vi "Unidirectional Quadrature Decoder.vi"(10 "B":bool, 11 "A":bool) -> (3 "Counter":i32)   [LabVIEW 2018]
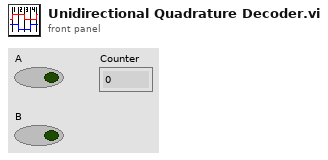
[diagram p1: front panel]
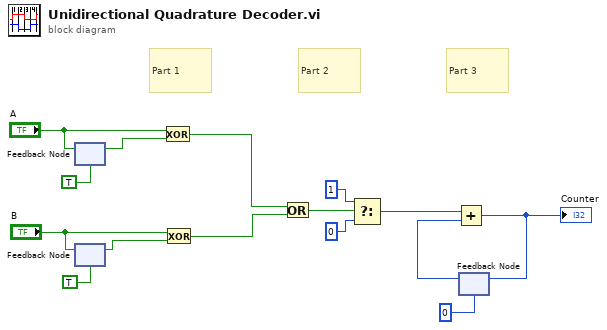
[diagram p0: block diagram]
diagram:
  # "Part 3"
  # "Part 2"
  # "Part 1"
  n1 = feedback-in #1("A") -> ()
  n2 = feedback #1(TRUE ("A")) -> (w7:bool)
  n3 = feedback #2(TRUE ("A")) -> (w5:bool)
  n4 = feedback-in #2("B") -> ()
  n5 = Exclusive Or(1:w7, 2:"A") -> (0:w15:bool)
  n6 = Exclusive Or(1:w5, 2:"B") -> (0:w14:bool)
  n7 = Or(x=w15, y=w14) -> (x .or. y?=w13:bool)
  n8 = Select(t=1, s=w13, f=0) -> (s? t:f=w9:i32)
  n9 = feedback #3(0) -> (w10:i32)
  n10 = Add(x=w9, y=w10) -> (x+y=w11:i32)
  "Counter" <- w11
  n11 = feedback-in #3(w11) -> ()
